vi "End Snap.vi"(8 "error in (no error)":errorcluster, 10 "Image out":T2, 11 "Refnum in":T1) -> (0 "error out":errorcluster)   [LabVIEW 2011]
uses:
  <vilib>/vision/Image Controls.llb/IMAQ Image.ctl
  <vilib>/userDefined/High Color/IMAQdx.ctl
  <vilib>/vision/driver/NI_Vision_Acquisition_Software.lvlib
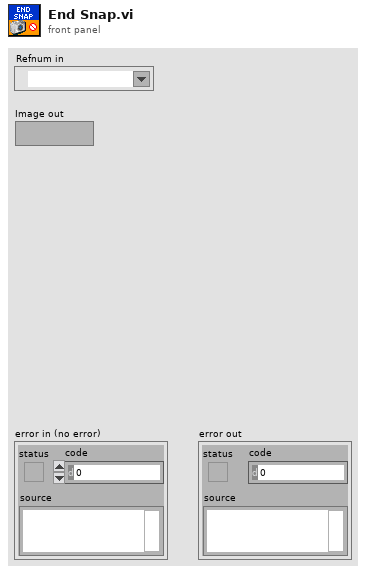
[diagram p1: front panel]
types:
  T1 = typedef "IMAQdx.ctl" = refnum<k21>
  T2 = typedef "IMAQ Image.ctl" = refnum<image>
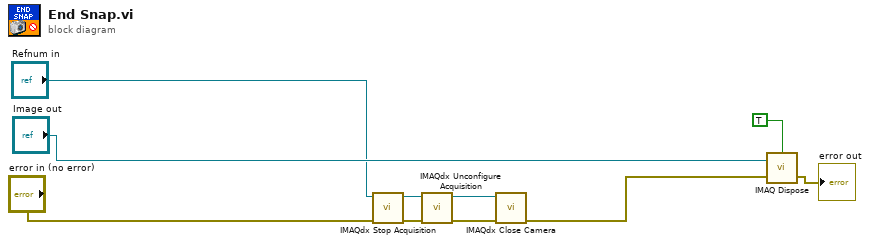
[diagram p0: block diagram]
diagram:
  n1 = call <vilib>:"IMAQdx Stop Acquisition.vi"("error in"="error in (no error)", "Session In"="Refnum in") -> ("error out"=w6:errorcluster, "Session Out"=w5:T1)  [unwired: 8 out]
  n2 = call <vilib>:"IMAQdx Unconfigure Acquisition.vi"("error in"=w6, "Session In"=w5) -> ("error out"=w7:errorcluster, "Session Out"=w8:T1)  [unwired: 8 out]
  n3 = call <vilib>:"IMAQdx Close Camera.vi"("error in"=w7, "Session In"=w8) -> ("error out"=w3:errorcluster)  [unwired: 9 out]
  n4 = call "IMAQ Dispose"("All Images? (No)"=TRUE, "Image"="Image out", "error in (no error)"=w3) -> ("error out"=→"error out":errorcluster)  [unwired: 3 in]
